vi "CloseByteStreamReference.vi"(1 "Byte Stream File Refnum":refnum<file>) -> (0 "error out":errorcluster)   [LabVIEW 2011]
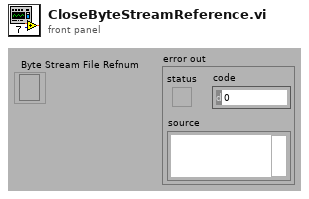
[diagram p1: front panel]
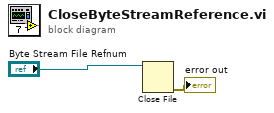
[diagram p0: block diagram]
diagram:
  n1 = Close File(refnum="Byte Stream File Refnum") -> (error out=→"error out":errorcluster)  [unwired: 1 in, 1 out]
